vi "Read queue reference.vi"(8 "error in (no error)":errorcluster, 11 "MockTransceiver in":refnum<class "MockTransceiver.lvclass">) -> (0 "error out":errorcluster, 2 "queue reference":refnum<queue>, 3 "MockTransceiver out":refnum<class "MockTransceiver.lvclass">)   [LabVIEW 2017, in "MockTransceiver.lvclass"]
uses:
  MockTransceiver.lvclass
  MockTransceiver.lvclass/MockTransceiver.ctl
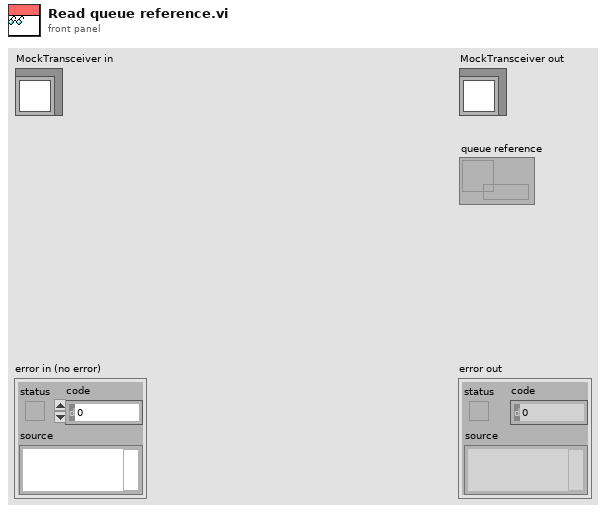
[diagram p1: front panel]
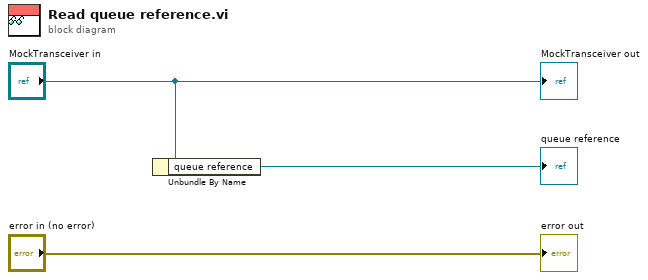
[diagram p0: block diagram]
diagram:
  n1 = Unbundle By Name("MockTransceiver in") -> ("queue reference"=→"queue reference":refnum<queue>)
  "error out" <- "error in (no error)"
  "MockTransceiver out" <- "MockTransceiver in"
